vi "Authenticate.vi"(8 "error in (no error)":errorcluster, 11 "Authentication in":refnum<class "Authentication.lvclass">) -> (0 "error out":errorcluster, 1 "User":string, 2 "Authenticated?":bool, 3 "Authentication out":refnum<class "Authentication.lvclass">)   [LabVIEW 2016, in "Authentication.lvclass"]
uses:
  Authentication.lvclass
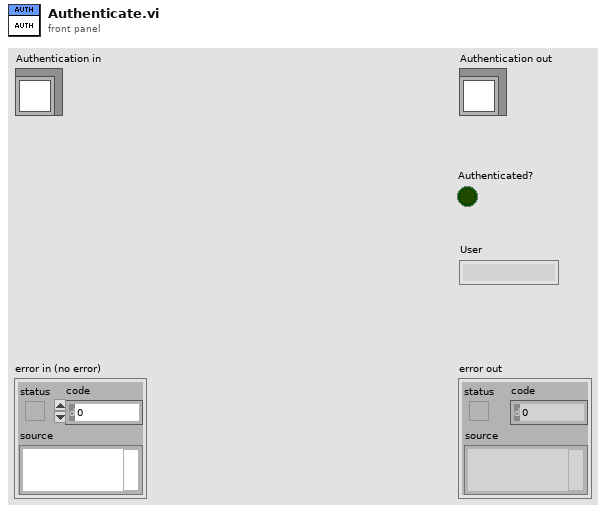
[diagram p1: front panel]
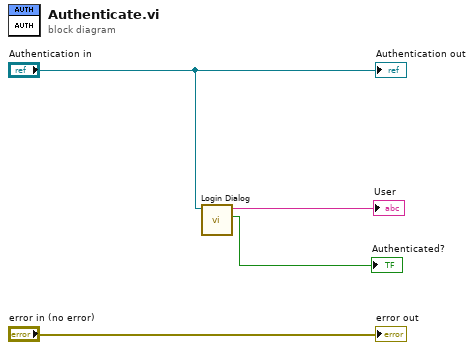
[diagram p0: block diagram]
diagram:
  n1 = call "Login Dialog.vi"("Authentication in"="Authentication in") -> ("Authenticated?"=→"Authenticated?":bool, "Username Out"=→"User":string)  [unwired: 9 in]
  "error out" <- "error in (no error)"
  "Authentication out" <- "Authentication in"
